vi "MultiplyTwoNumbers.vi"(10 "Number 2":dbl, 11 "Number 1":dbl) -> (3 "Product":dbl)   [LabVIEW 2015]
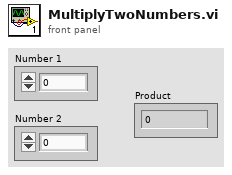
[diagram p1: front panel]
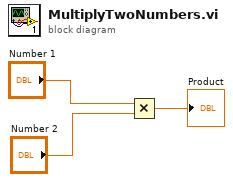
[diagram p0: block diagram]
diagram:
  n1 = Multiply(x="Number 1", y="Number 2") -> (x*y=→"Product":dbl)
